vi "Sub_CalculateNormalizedLinearFcnOutput.vi"(1 "Saturate to 0-1 ?":bool, 2 "B coefficient":dbl, 3 "A coefficient":dbl, 4 "Value":dbl) -> (0 "Normalized value":dbl)   [LabVIEW 2021]
doc: "This subVI serves a function to calculate an output from linear function of defined y = Ax + B, A,B being defined as required inputs, as well as x. This subVI allows also to verify whether output fits to [0,1] range, and if needed (optional) it can also saturate the output to be 0 if y < 0 and 1 if y > 1."
panel:
  # "Inputs:"
  # "Outputs:"
  # "Required:"
  # "Optional:"
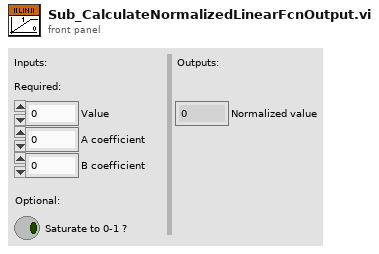
[diagram p1: front panel]
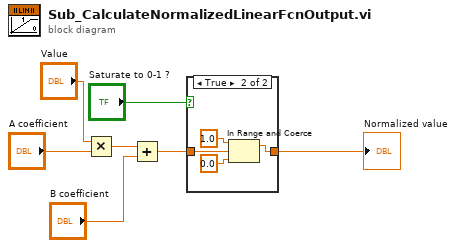
[diagram p0: block diagram]
diagram:
  n1 = Multiply(x="Value", y="A coefficient") -> (x*y=w5:dbl)
  n2 = Add(x=w5, y="B coefficient") -> (x+y=w3:dbl)
  n3 = case shown="True" "Saturate to 0-1 ?" {
    tunnel: w3 -> [w8 w12]
    tunnel: [w8 w9] -> w1
    frame False {
    }
    frame True {
      n4 = In Range and Coerce(upper limit=1.0, x=w12, lower limit=0.0) -> (coerced(x)=w9:dbl)  [unwired: 1 out]
    }
  }
  "Normalized value" <- w1
